vi "Parameter (Channel).vi"(8 "error in (no error)":errorcluster, 11 "Node Ptr":T1 format="%.0x") -> (0 "error out":errorcluster)   [LabVIEW 2020, in "Communication Bus Template System Explorer.lvlib" / "Implementation.lvlib"]
uses:
  Implementation.lvlib
  <vilib>/NI VeriStand/Custom Device API/Custom Device Item Ref.ctl
  <vilib>/NI VeriStand/Custom Device API/Custom Device API.lvlib
  Scripting/Communication Bus Template Scripting.lvlib
  Protocol/Implementations/ARINC429/ARINC429-32bit/32-bit Word.lvclass
panel:
  out "Default Value (Raw Bits)":u32 format="%032b"
  out "TiggerDValChange":bool
  in  "Unit":string
  in  "Encoding Type":enum16{"BNR", "BCD", "Discrete"}(ring)
  in  "Scale Offset":dbl format="%#_6f"
  in  "Scale Factor":dbl format="%#_6f"
  in  "Signed?":bool
  in  "Default Value (Scaled)":dbl
  in  "Number of Bits":i32=1 min=1 max=32
  in  "Start Bit":i32=1
  in  "SHDocVw.IWebBrowser":refnum<k7>(container)
  in  "Specific Header":cluster{"Section Name":string}={"Section Name"="Specific Page Settings"}
  in  "General Header":cluster{"Section Name":string}={"Section Name"="General Page Settings"}
  in  "Description":string
  in  "Name":string
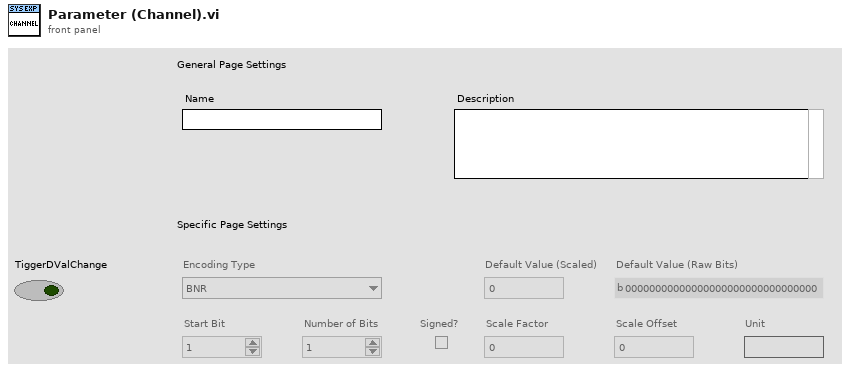
[diagram p1: front panel]
types:
  T1 = typedef "Custom Device API.lvlib/Custom Device Item Ref.ctl" = u64
  T2 = typedef "Custom Device API.lvlib/Custom Device Channel.ctl" = cluster{"Type":T3, "Units":string, "Default Value":dbl, "Faultable":bool, "Scalable":bool}
  T3 = typedef "Custom Device API.lvlib/Custom Device Channel Type.ctl" = enum16{"Input", "Output"}
  T4 = typedef "Custom Device API.lvlib/Custom Device Commands.ctl" = enum16{"Default", "Item renamed", "Shutdown", "Dynamic button pressed"}
  T5 = typedef "Custom Device API.lvlib/Custom Device Item Info.ctl" = cluster{"Name":string, "Is Channel":bool, "GUID":string, "Is Waveform":bool}
  T6 = typedef "ARINC 429.lvclass/Parameter Definition.ctl" = cluster{"start index":i32, "size":i32, "encoding":T7, "signed":bool, "scale multiplier":dbl, "scale offset":dbl}
  T7 = typedef "Encoding and Decoding.lvlib/Encoding.ctl" = enum16{"BNR", "BCD", "Discrete"}
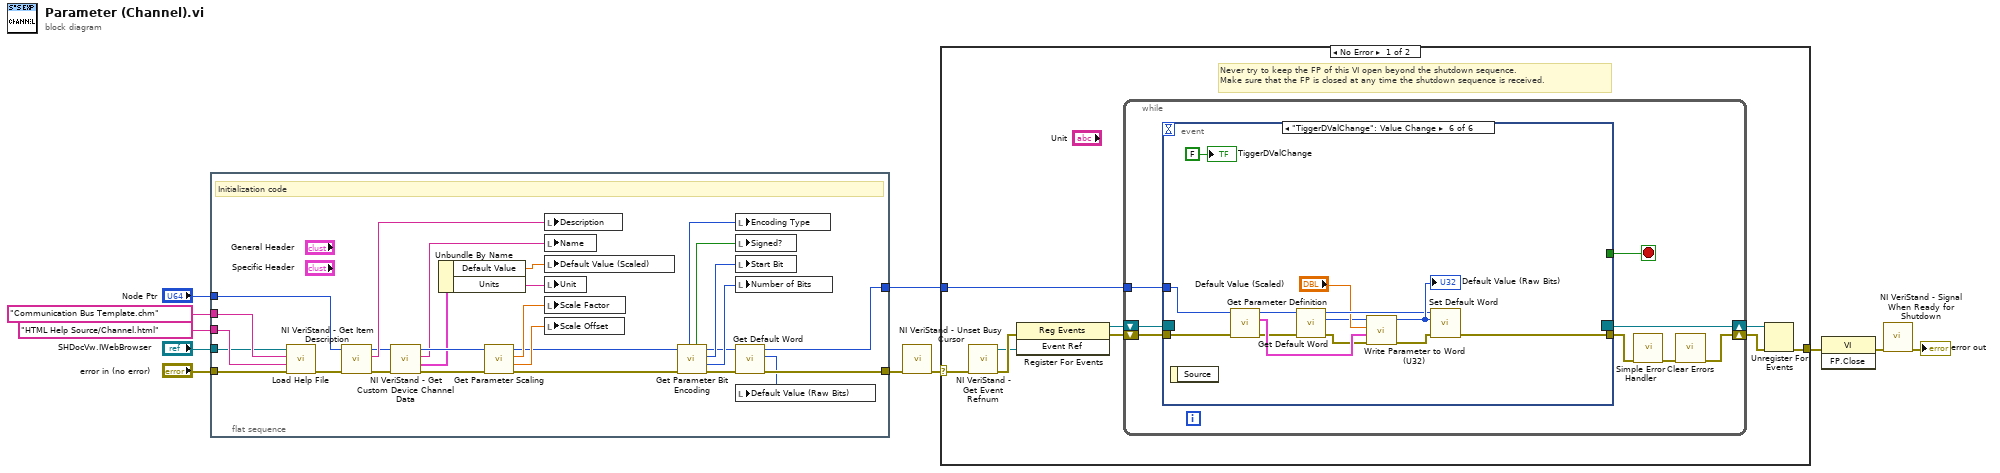
[diagram p0: block diagram]
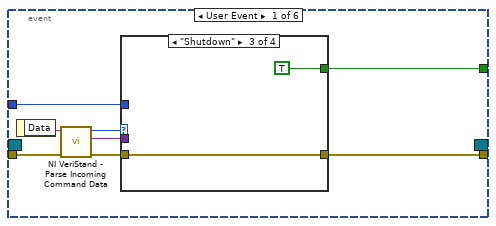
[diagram p2: hidden frame]
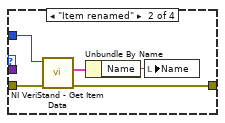
[diagram p4: hidden frame]
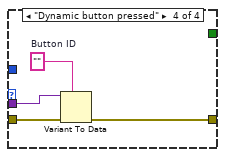
[diagram p5: hidden frame]
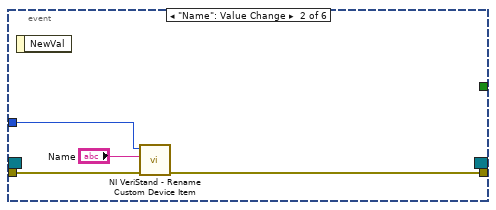
[diagram p6: hidden frame]
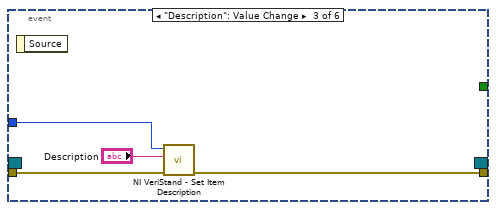
[diagram p7: hidden frame]
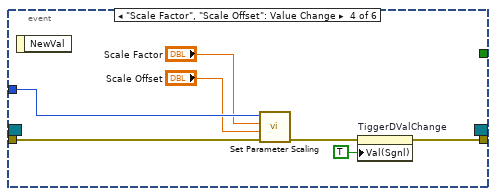
[diagram p8: hidden frame]
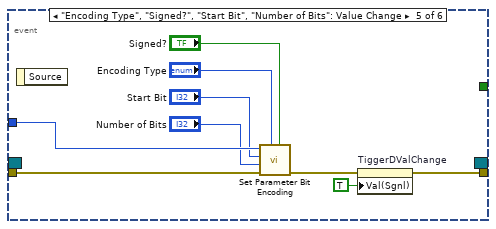
[diagram p9: hidden frame]
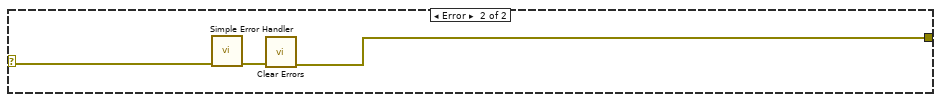
[diagram p10: hidden frame]
diagram:
  n1 = flat-sequence "Initialization code" {
    tunnel: "error in (no error)" -> [w37]
    tunnel: "Node Ptr" -> [w39]
    tunnel: [w14] -> w7
    tunnel: "SHDocVw.IWebBrowser" -> [w33]
    tunnel: "HTML Help Source/Channel.html" ("CD_CHM_Section") -> [w35]
    tunnel: "Communication Bus Template.chm" ("CD_CHM_FileName") -> [w34]
    tunnel: [w13] -> w1
    frame #0 {
      # "Initialization code"
      n2 = call "Load Help File.vi"("error in (no error)"=w37, "HTML File to Load"=w35, "Main CHM File"=w34, "Browser"=w33) -> ("error out"=w36:errorcluster)  [unwired: 7 in]
      n3 = call <vilib>:"NI VeriStand - Get Item Description.vi"("error in (no error)"=w36, "Item Ref in"=w39) -> ("error out"=w29:errorcluster, "Description"=w38:string, "Item Ref out"=w30:T1)  [unwired: 7 out]
      n4 = call <vilib>:"NI VeriStand - Get Custom Device Channel Data.vi"("error in (no error)"=w29, "Channel Ref in"=w30) -> ("error out"=w28:errorcluster, "Channel"=w25:T2, "Channel Name"=w26:string, "Channel Ref out"=w27:T1)  [unwired: 4 in, 2 out]
      n5 = Unbundle By Name(w25) -> ("Default Value"=w24:dbl, "Units"=w17:string)
      n6 = call "Get Parameter Scaling.vi"("error in (no error)"=w28, "Item Ref in"=w27) -> ("error out"=w22:errorcluster, "scale offset"=w31:dbl, "scale multiplier"=w32:dbl, "Item Ref out"=w23:T1)  [unwired: 6 in]
      n7 = local write "Description"(w38) -> ()
      n8 = local write "Name"(w26) -> ()
      n9 = local write "Default Value (Scaled)"(w24) -> ()
      n10 = local write "Unit"(w17) -> ()
      n11 = local write "Scale Factor"(w32) -> ()
      n12 = local write "Scale Offset"(w31) -> ()
      n13 = call "Get Parameter Bit Encoding.vi"("error in"=w22, "Item Ref in"=w23) -> ("error out"=w15:errorcluster, "number of bits"=w18:i32, "start bit"=w19:i32, "Item Ref out"=w16:T1, "signed?"=w20:bool, "encoding type"=w21:enum16{"BNR", "BCD", "Discrete"})  [unwired: 4 in]
      n14 = local write "Encoding Type"(w21) -> ()
      n15 = local write "Signed?"(w20) -> ()
      n16 = local write "Start Bit"(w19) -> ()
      n17 = local write "Number of Bits"(w18) -> ()
      n18 = call "Get Default Word.vi"("error in"=w15, "Item Ref in"=w16) -> ("error out"=w14:errorcluster, "default word"=w12:u32, "Item Ref out"=w13:T1)  [unwired: 7 in]
      n19 = local write "Default Value (Raw Bits)"(w12) -> ()
    }
  }
  n20 = call <vilib>:"NI VeriStand - Unset Busy Cursor.vi"("error in (no error)"=w7) -> ("error out"=w6:errorcluster)  [unwired: 10 out]
  n21 = case shown="No Error" w6 {
    selector: w6 -> [w40 w116]
    tunnel: [w45 w114] -> w11
    tunnel: w1 -> [w41 _]
    frame No Error {
      # "Never try to keep the FP of this VI open beyond the shutdown sequence.\nMake sure that the FP is closed at any time the shutdown sequence is received."
      n22 = call <vilib>:"NI VeriStand - Get Event Refnum.vi"("error in (no error)"=w40) -> ("error out"=w48:errorcluster, "Event Ref"=w44:refnum<user-event>)  [unwired: 9 out]
      n23 = register-events(error in=w48, w44) -> (reference out=w42:refnum<event-registration>, error out=w43:errorcluster)  [unwired: 1 in]
      n24 = while {
        tunnel: w41 -> [w52]
        shift-right: [w49] -> w46
        shift-left: w43 -> [w55]
        shift-right: [w56] -> w47
        shift-left: w42 -> [w54]
        stop <- w53 stop-if-true
        n25 = event shown="[5] \"TiggerDValChange\": Value Change" {
          selector: w54 -> [_ _ _ _ _ _]
          dyn-events: [_ _ _ _ _ _] -> w56
          timeout: _ -> [_ _ _ _ _ _]
          tunnel: w55 -> [w64 w80 w83 w90 w99 w105]
          tunnel: [w60 _ _ _ _ _] -> w53
          tunnel: [w59 w79 w82 w86 w93 w112] -> w51
          tunnel: w52 -> [w58 w78 w84 w91 w100 w106]
          event User Event {
            n26 = event-data() -> ("Data"=w63:string)  [unwired: 1 out]
            n27 = call <vilib>:"NI VeriStand - Parse Incoming Command Data.vi"("error in (no error)"=w64, "Incoming data"=w63) -> ("error out"=w62:errorcluster, "Outgoing data"=w57:variant, "Action"=w61:T4)  [unwired: 7 out]
            n28 = case shown="\"Shutdown\"" w61 {
              tunnel: w62 -> [w65 w70 w71 w76]
              tunnel: [_ _ TRUE _] -> w60
              tunnel: [w65 w67 w71 w73] -> w59
              tunnel: w58 -> [_ w69 _ _]
              tunnel: w57 -> [_ _ _ w75]
              frame "Default", Default {
              }
              frame "Item renamed" {
                n29 = call <vilib>:"NI VeriStand - Get Item Data.vi"("error in (no error)"=w70, "Item Ref in"=w69) -> ("error out"=w67:errorcluster, "Item Info"=w68:T5)  [unwired: 8 out]
                n30 = Unbundle By Name(w68) -> ("Name"=w66:string)
                n31 = local write "Name"(w66) -> ()
              }
              frame "Shutdown" {
              }
              frame "Dynamic button pressed" {
                w74 = ""  # Button ID
                n32 = Variant To Data(error in=w76, type=w74, Variant=w75) -> (error out=w73:errorcluster)  [unwired: 1 out]
              }
            }
          }
          event "Name": Value Change {
            n33 = event-data() -> ()  [unwired: 2 out]
            n34 = call <vilib>:"NI VeriStand - Rename Custom Device Item.vi"("error in (no error)"=w80, "New Name"="Name", "Item Ref in"=w78) -> ("error out"=w79:errorcluster)  [unwired: 1 in, 7 out]
          }
          event "Description": Value Change {
            n35 = event-data() -> ()  [unwired: 2 out]
            n36 = call <vilib>:"NI VeriStand - Set Item Description.vi"("error in (no error)"=w83, "Description"="Description", "Item Ref in"=w84) -> ("error out"=w82:errorcluster)  [unwired: 8 out]
          }
          event "Scale Factor", "Scale Offset": Value Change {
            n37 = event-data() -> ()  [unwired: 2 out]
            n38 = call "Set Parameter Scaling.vi"("error in (no error)"=w90, "scale offset"="Scale Offset", "scale multiplier"="Scale Factor", "Item Ref in"=w91) -> ("error out"=w87:errorcluster)  [unwired: 6 in, 1 out]
            n39 = property on="TiggerDValChange" class="Bool (strict)"(error in=w87, "Val(Sgnl)"=TRUE ("Value (Signaling)")) -> (error out=w86:errorcluster)  [unwired: 1 in, 1 out]
          }
          event "Encoding Type", "Signed?", "Start Bit", "Number of Bits": Value Change {
            n40 = event-data() -> ()  [unwired: 2 out]
            n41 = call "Set Parameter Bit Encoding.vi"("signed?"="Signed?", "encoding"="Encoding Type", "error in"=w99, "number of bits"="Number of Bits", "start bit"="Start Bit", "Item Ref in"=w100) -> ("error out"=w94:errorcluster)  [unwired: 4 in, 1 out]
            n42 = property on="TiggerDValChange" class="Bool (strict)"(error in=w94, "Val(Sgnl)"=TRUE ("Value (Signaling)")) -> (error out=w93:errorcluster)  [unwired: 1 in, 1 out]
          }
          event "TiggerDValChange": Value Change {
            n43 = event-data() -> ()  [unwired: 2 out]
            n44 = call "Get Parameter Definition.vi"("error in"=w105, "parameter ref in"=w106) -> ("error out"=w107:errorcluster, "parameter definition out"=w109:T6, "parameter ref out"=w108:T1)  [unwired: 7 in]
            n45 = call "Get Default Word.vi"("error in"=w107, "Item Ref in"=w108) -> ("error out"=w104:errorcluster, "default word"=w101:u32, "Item Ref out"=w103:T1)  [unwired: 7 in]
            n46 = call "Write Parameter to Word (U32).vi"("error in"=w104, "parameter definition in"=w109, "scaled data"="Default Value (Scaled)", "32-bit word in"=w101) -> ("error out"=w111:errorcluster, "32-bit word out"=w110:u32)  [unwired: 6 in]
            "Default Value (Raw Bits)" <- w110
            n47 = call "Set Default Word.vi"("error in"=w111, "default word"=w110, "Item Ref in"=w103) -> ("error out"=w112:errorcluster)  [unwired: 7 in, 1 out]
            "TiggerDValChange" <- FALSE ("TiggerDValChange")
          }
        }
        n48 = call <vilib>:"Simple Error Handler.vi"("error in (no error)"=w51) -> ("error out"=w50:errorcluster)  [unwired: 1 in, 7 out]
        n49 = call <vilib>:"Clear Errors.vi"("error in (no error)"=w50) -> ("error out"=w49:errorcluster)  [unwired: 1 in, 5 out]
      }
      n50 = Unregister For Events(event registration refnum=w47, error in=w46) -> (error out=w45:errorcluster)
    }
    frame Error {
      n51 = call <vilib>:"Simple Error Handler.vi"("error in (no error)"=w116) -> ("error out"=w115:errorcluster)  [unwired: 1 in, 7 out]
      n52 = call <vilib>:"Clear Errors.vi"("error in (no error)"=w115) -> ("error out"=w114:errorcluster)  [unwired: 1 in, 5 out]
    }
  }
  n53 = invoke class="VI" method="FP.Close"(error in=w11) -> (error out=w10:errorcluster)  [unwired: 2 in, 2 out]
  n54 = call <vilib>:"NI VeriStand - Signal When Ready for Shutdown.vi"("error in (no error)"=w10) -> ("error out"=→"error out":errorcluster)  [unwired: 10 out]
